vi "Part 2.vi"(11 "Input":string) -> (3 "Output":i64)   [LabVIEW 2021]
panel:
  out "Unknowns scanners left":i32
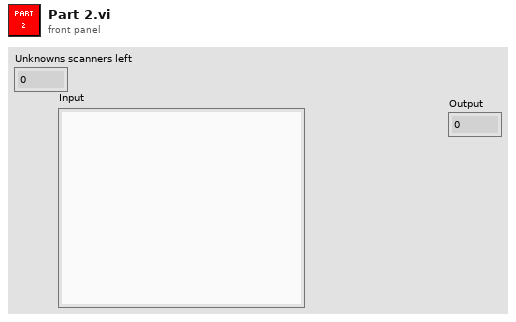
[diagram p1: front panel]
types:
  T1 = cluster{"Beacons":cluster{"X":i64, "Y":i64, "Z":i64}[]}[]
  T2 = cluster{"Beacons":cluster{"X":i64, "Y":i64, "Z":i64}[]}
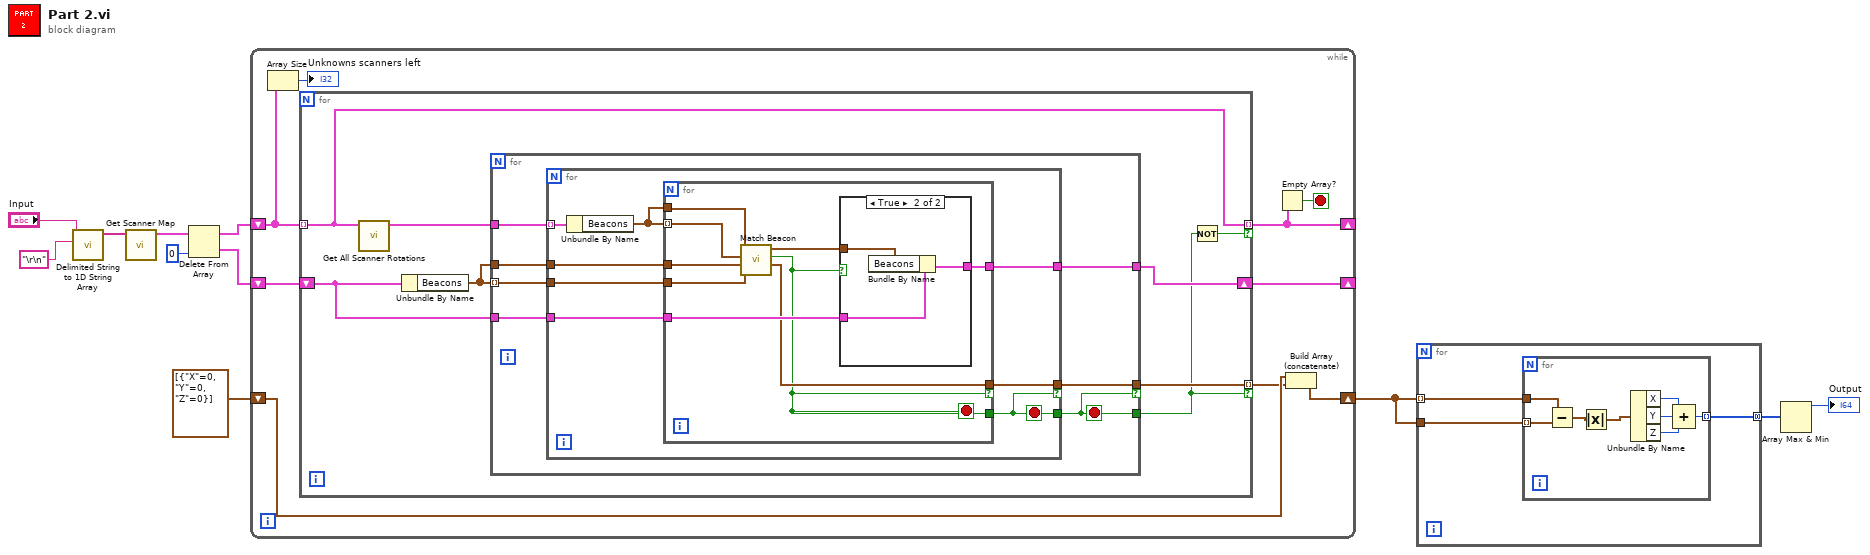
[diagram p0: block diagram]
diagram:
  n1 = call <vilib>:"Delimited String to 1D String Array.vi"("delimiter"="\r\n", "delimited string"="Input") -> ("string array"=w10:string[])  [unwired: 9 in]
  n2 = call "Get Scanner Map.vi"("Input"=w10) -> ("Scanners"=w8:T1)  [unwired: 10 in]
  n3 = Delete From Array(array=w8, index=0) -> (deleted portion=w6:T2, array with subset deleted=w7:T1)  [unwired: 1 in]
  n4 = while {
    shift-right: [w19] -> _
    shift-left: w6 -> [w20]
    shift-right: [w18] -> _
    shift-left: w7 -> [w16]
    shift-right: [w12] -> w3
    shift-left: cluster{"X":i64, "Y":i64, "Z":i64}[] [{"X"=0, "Y"=0, "Z"=0}] ("Array") -> [w14]
    stop <- w17 stop-if-true
    n5 = Array Size(array=w16) -> (size(s)=→"Unknowns scanners left":i32)
    n6 = for {
      tunnel: w16 -> [w27] mode=indexing
      shift-right: [w24] -> w19
      shift-left: w20 -> [w23]
      tunnel: [w27] -> w18 mode=indexing if=w28
      tunnel: [w22] -> w13 mode=indexing if=w21
      n7 = call "Get All Scanner Rotations.vi"("Scanner"=w27) -> ("Scanner Rotations"=w26:T1)  [unwired: 10 in]
      n8 = Unbundle By Name(w23) -> ("Beacons"=w25:cluster{"X":i64, "Y":i64, "Z":i64}[])
      n9 = for {
        tunnel: [w29] -> w21
        tunnel: w26 -> [w34]
        tunnel: w25 -> [w35] mode=indexing
        tunnel: w25 -> [w33]
        tunnel: [w32] -> w24
        tunnel: w23 -> [w31]
        tunnel: [w30] -> w22 if=w29
        stop <- w29 stop-if-true
        n10 = for {
          tunnel: [w36] -> w29
          tunnel: w35 -> [w43]
          tunnel: w34 -> [w40] mode=indexing
          tunnel: w33 -> [w41]
          tunnel: [w39] -> w32
          tunnel: w31 -> [w38]
          tunnel: [w37] -> w30 if=w36
          stop <- w36 stop-if-true
          n11 = Unbundle By Name(w40) -> ("Beacons"=w42:cluster{"X":i64, "Y":i64, "Z":i64}[])
          n12 = for {
            tunnel: w43 -> [w47]
            tunnel: w42 -> [w49] mode=indexing
            tunnel: w42 -> [w50]
            tunnel: w41 -> [w48]
            tunnel: w38 -> [w51]
            tunnel: [w52] -> w39
            tunnel: [w44] -> w36
            tunnel: [w45] -> w37 if=w44
            stop <- w44 stop-if-true
            n13 = call "Match Beacon.vi"("Known Beacon"=w47, "Known Beacons"=w48, "Unknown Beacon"=w49, "Unknown Beacons"=w50) -> ("Scanner Position"=w45:cluster{"X":i64, "Y":i64, "Z":i64}, "Match?"=w44:bool, "New Beacons"=w46:cluster{"X":i64, "Y":i64, "Z":i64}[])  [unwired: 5 in]
            n14 = case shown="True" w44 {
              tunnel: [w53 w55] -> w52
              tunnel: w51 -> [w53 w56]
              tunnel: w46 -> [_ w54]
              frame False {
              }
              frame True {
                n15 = Bundle By Name(cluster=w56, "Beacons"=w54) -> (w55:T2)
              }
            }
          }
        }
      }
      n16 = Not(x=w21) -> (.not. x?=w28:bool)
    }
    n17 = Empty Array?(array=w18) -> (empty?=w17:bool)
    n18 = Build Array (concatenate)(w14, w13) -> (w12:cluster{"X":i64, "Y":i64, "Z":i64}[])
  }
  n19 = for {
    tunnel: w3 -> [w58] mode=indexing
    tunnel: w3 -> [w59]
    tunnel: [w57] -> w2 mode=concatenating
    n20 = for {
      tunnel: w59 -> [w66] mode=indexing
      tunnel: w58 -> [w67]
      tunnel: [w60] -> w57 mode=indexing
      n21 = Subtract(x=w67, y=w66) -> (x-y=w65:cluster{"X":i64, "Y":i64, "Z":i64})
      n22 = Absolute Value(x=w65) -> (abs(x)=w64:cluster{"X":i64, "Y":i64, "Z":i64})
      n23 = Unbundle By Name(w64) -> ("X"=w62:i64, "Y"=w63:i64, "Z"=w61:i64)
      n24 = Compound Arithmetic op=ADD(w62, w63, w61) -> (w60:i64)
    }
  }
  n25 = Array Max & Min(array=w2) -> (max value=→"Output":i64)  [unwired: 3 out]
